vi "initializer_output.vi"(0 "Run":refnum<vi>, 1 "Endtime":refnum<vi>, 2 "Refresh Button":refnum<vi>, 3 "Starttime":refnum<vi>, 4 "Load Simulation File":refnum<vi>, 5 "Parameters Tree":refnum<vi>, 6 "Save Specs":refnum<vi>, 7 "Load Spec File":refnum<vi>, 8 "Dataflow Out":refnum<vi>, 9 "Load Vali File":refnum<vi>, 10 "Validate":refnum<vi>, 11 "Cancel Button":refnum<vi>) -> (14 "Run?":bool)   [LabVIEW 2019]
uses:
  lib/libSimulationControl/libSimulationControl.lvlib
panel:
  # "*******************************************************************\nBiogas Plant Control\n\nAuthor: Paul Zügel\nGCSC-Frankfurt am Main 2020\n\n*******************************************************************"
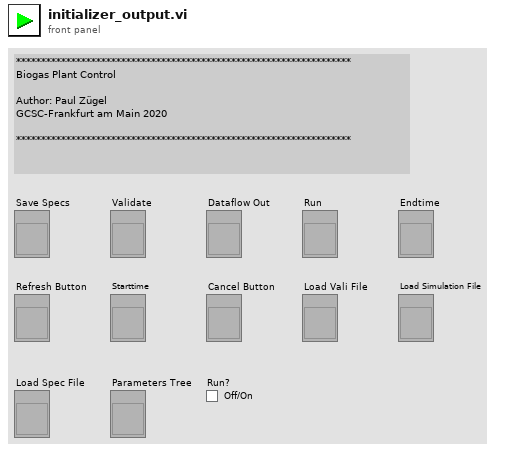
[diagram p1: front panel]
types:
  T1 = enum8{"Enabled", "Disabled", "Disabled and Grayed Out"}
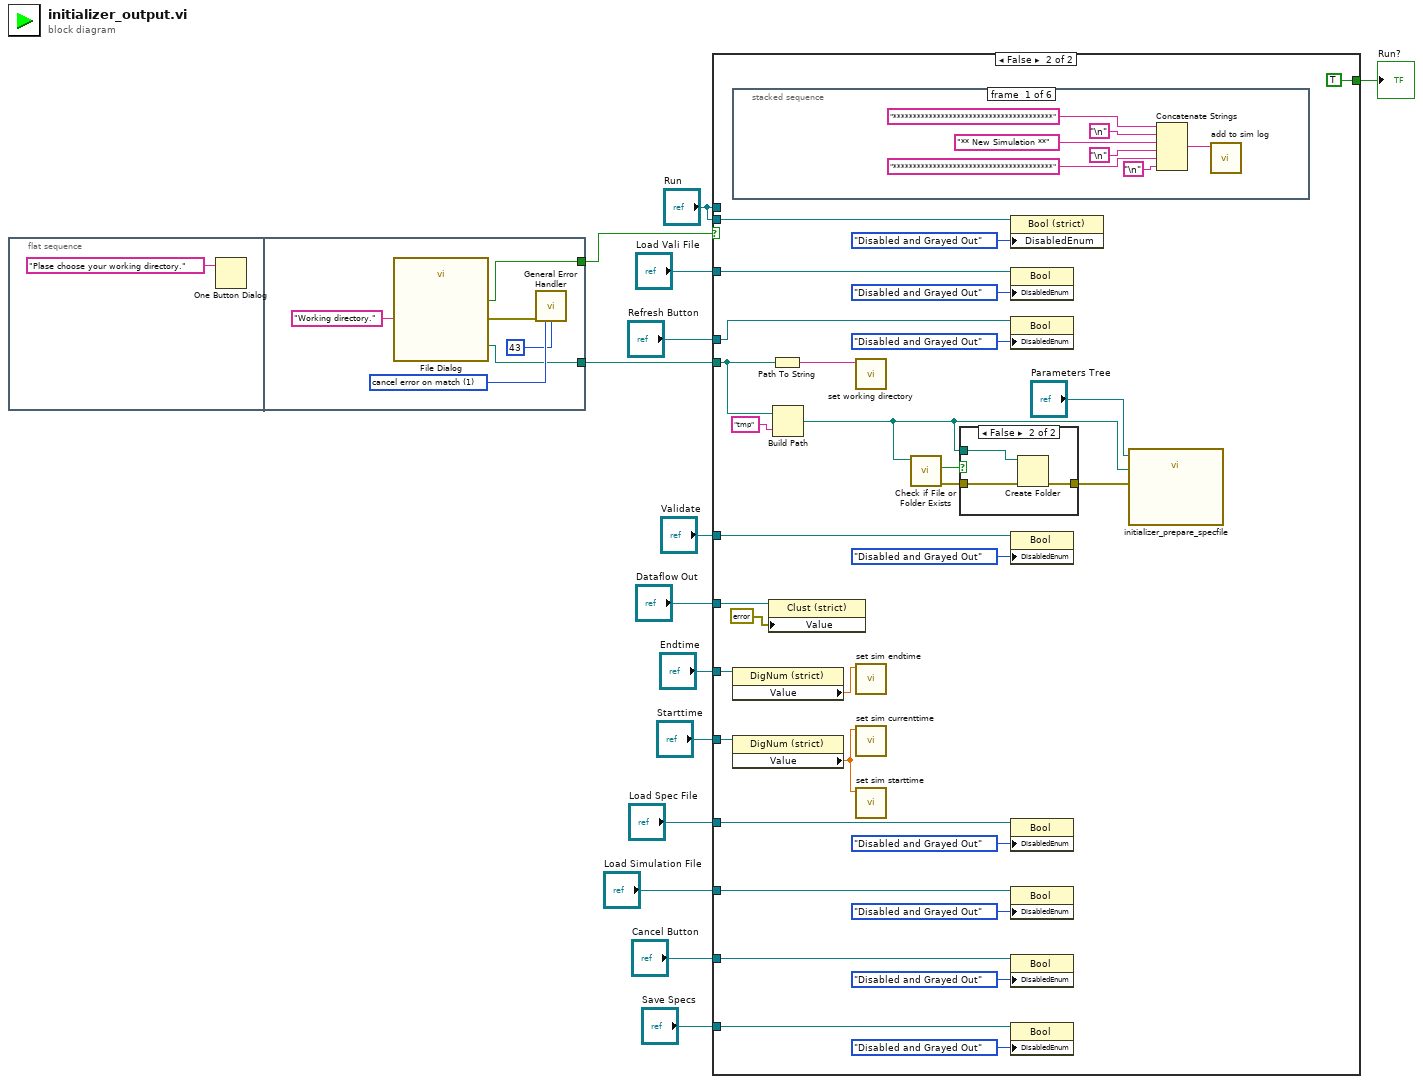
[diagram p0: block diagram]
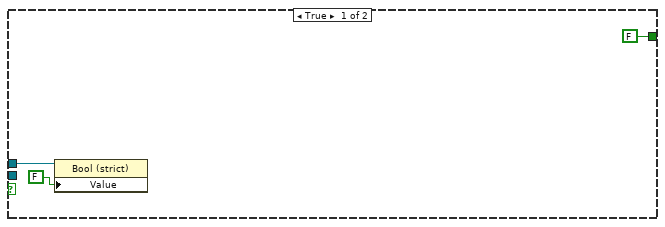
[diagram p2: hidden frame]
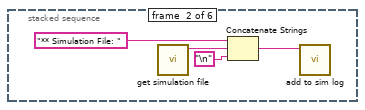
[diagram p3: hidden frame]
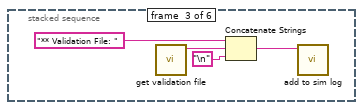
[diagram p4: hidden frame]
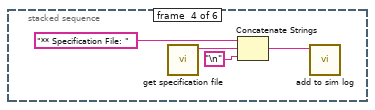
[diagram p5: hidden frame]
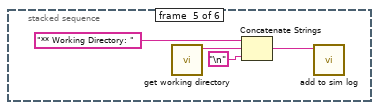
[diagram p6: hidden frame]
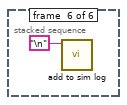
[diagram p7: hidden frame]
diagram:
  n1 = flat-sequence {
    tunnel: [w21] -> w12
    tunnel: [w16] -> w14
    frame #0 {
      n2 = One Button Dialog(message="Plase choose your working directory.") -> ()  [unwired: 1 in, 1 out]
    }
    frame #1 {
      w18 = 1 items=["no exception", "cancel error on match", "set error on match"] ("[exception action] (none:0)")
      n3 = call "File Dialog"("prompt"="Working directory.") -> ("selected path"=w16:path, "cancelled"=w21:bool, "error out"=w19:errorcluster)  [unwired: 11 in, 1 out]
      n4 = call <vilib>:"General Error Handler.vi"("error in (no error)"=w19, "[exception action] (none:0)"=w18, "[exception code]"=43) -> ()  [unwired: 8 in, 5 out]
    }
  }
  n5 = case shown="False" w12 {
    tunnel: [FALSE TRUE] -> w13
    tunnel: w14 -> [_ w46]
    tunnel: "Run" -> [w22 _]
    tunnel: "Run" -> [_ w39]
    tunnel: "Validate" -> [_ w38]
    tunnel: "Save Specs" -> [_ w37]
    tunnel: "Refresh Button" -> [_ w36]
    tunnel: "Load Simulation File" -> [_ w35]
    tunnel: "Load Spec File" -> [_ w34]
    tunnel: "Load Vali File" -> [_ w33]
    tunnel: "Cancel Button" -> [_ w32]
    tunnel: "Starttime" -> [_ w31]
    tunnel: "Endtime" -> [_ w30]
    tunnel: "Dataflow Out" -> [_ w29]
    frame True {
      n6 = property on="Property Node" class="Bool (strict)"(reference=w22, "Value"=FALSE ("Run")) -> ()  [unwired: 1 in, 2 out]
    }
    frame False {
      n7 = stacked-sequence {
        frame #0 {
          n8 = Concatenate Strings("****************************************" ("string"), "\n", "** New Simulation **" ("string"), "\n", "****************************************" ("string"), "\n") -> (w62:string)
          n9 = call "add to sim log.vi"("log"=w62) -> ()  [unwired: 10 in, 1 out]
        }
        frame #1 {
          n10 = call "get simulation file.vi"() -> ("function return"=w66:string)  [unwired: 10 in, 1 out]
          n11 = Concatenate Strings("** Simulation File: " ("string"), w66, "\n") -> (w65:string)
          n12 = call "add to sim log.vi"("log"=w65) -> ()  [unwired: 10 in, 1 out]
        }
        frame #2 {
          n13 = call "get validation file.vi"() -> ("function return"=w70:string)  [unwired: 10 in, 1 out]
          n14 = Concatenate Strings("** Validation File: " ("string"), w70, "\n") -> (w69:string)
          n15 = call "add to sim log.vi"("log"=w69) -> ()  [unwired: 10 in, 1 out]
        }
        frame #3 {
          n16 = call "get specification file.vi"() -> ("function return"=w74:string)  [unwired: 10 in, 1 out]
          n17 = Concatenate Strings("** Specification File: " ("string"), w74, "\n") -> (w73:string)
          n18 = call "add to sim log.vi"("log"=w73) -> ()  [unwired: 10 in, 1 out]
        }
        frame #4 {
          n19 = call "get working directory.vi"() -> ("function return"=w78:string)  [unwired: 10 in, 1 out]
          n20 = Concatenate Strings("** Working Directory: " ("string"), w78, "\n") -> (w77:string)
          n21 = call "add to sim log.vi"("log"=w77) -> ()  [unwired: 10 in, 1 out]
        }
        frame #5 {
          n22 = call "add to sim log.vi"("log"="\n") -> ()  [unwired: 10 in, 1 out]
        }
      }
      n23 = property class="DigNum (strict)"(reference=w30) -> ("Value"=w43:dbl)  [unwired: 1 in, 2 out]
      n24 = property class="DigNum (strict)"(reference=w31) -> ("Value"=w42:dbl)  [unwired: 1 in, 2 out]
      n25 = property class="Clust (strict)"(reference=w29, "Value"=errorcluster {"status"=FALSE, "code"=0, "source"=""} ("error constant")) -> ()  [unwired: 1 in, 2 out]
      n26 = Path To String(path=w46) -> (string=w41:string)
      n27 = Build Path(base path=w46, name or relative path="tmp") -> (appended path=w26:path)
      n28 = call "set working directory.vi"("dir"=w41) -> ()  [unwired: 10 in, 1 out]
      n29 = call "set sim endtime.vi"("time"=w43) -> ()  [unwired: 10 in, 1 out]
      n30 = call "set sim currenttime.vi"("time"=w42) -> ()  [unwired: 10 in, 1 out]
      n31 = call "set sim starttime.vi"("time"=w42) -> ()  [unwired: 10 in, 1 out]
      n32 = call <vilib>:"Check if File or Folder Exists.vi"("path"=w26) -> ("error out"=w27:errorcluster, "file or folder exists?"=w44:bool)  [unwired: 8 in, 1 out]
      n33 = case shown="False" w44 {
        tunnel: w26 -> [_ w83]
        tunnel: [w80 w82] -> w28
        tunnel: w27 -> [w80 w81]
        frame True {
        }
        frame False {
          n34 = Create Folder(path (use dialog)=w83, error in=w81) -> (error out=w82:errorcluster)  [unwired: 1 in, 2 out]
        }
      }
      n35 = property on="Property Node" class="Bool (strict)"(reference=w39, "DisabledEnum"=T1."Disabled and Grayed Out" ("Disabled")) -> ()  [unwired: 1 in, 2 out]
      n36 = property on="Property Node" class="Bool"(reference=w33, "DisabledEnum"=T1."Disabled and Grayed Out" ("Disabled")) -> ()  [unwired: 1 in, 2 out]
      n37 = property on="Property Node" class="Bool"(reference=w36, "DisabledEnum"=T1."Disabled and Grayed Out" ("Disabled")) -> ()  [unwired: 1 in, 2 out]
      n38 = property on="Property Node" class="Bool"(reference=w38, "DisabledEnum"=T1."Disabled and Grayed Out" ("Disabled")) -> ()  [unwired: 1 in, 2 out]
      n39 = property on="Property Node" class="Bool"(reference=w34, "DisabledEnum"=T1."Disabled and Grayed Out" ("Disabled")) -> ()  [unwired: 1 in, 2 out]
      n40 = property on="Property Node" class="Bool"(reference=w35, "DisabledEnum"=T1."Disabled and Grayed Out" ("Disabled")) -> ()  [unwired: 1 in, 2 out]
      n41 = property on="Property Node" class="Bool"(reference=w32, "DisabledEnum"=T1."Disabled and Grayed Out" ("Disabled")) -> ()  [unwired: 1 in, 2 out]
      n42 = property on="Property Node" class="Bool"(reference=w37, "DisabledEnum"=T1."Disabled and Grayed Out" ("Disabled")) -> ()  [unwired: 1 in, 2 out]
      n43 = call "initializer_prepare_specfile.vi"("error in (no error)"=w28, "appended path"=w26, "TreeControl in"="Parameters Tree") -> ()  [unwired: 9 in]
    }
  }
  "Run?" <- w13
